vi "DAQ-WriteReadSine.vi"(0 "Maximum Input":dbl, 1 "Minimum Input":dbl, 5 "Physical Input Channel":tag, 7 "tiempo (s)":dbl, 9 "Amplitud":dbl, 11 "Frecuencia":dbl, 12 "Fs (S/s)":dbl, 13 "Minimum Output":dbl, 14 "Maximum Output":dbl, 15 "Physical Output Channel":tag) -> (4 "Vout":dbl, 6 "Output":dbl[](graph), 8 "Vin":dbl, 10 "Input":dbl[](graph))   [LabVIEW 2010]
uses:
  <vilib>/Utility/error.llb/DialogType.ctl
  <vilib>/DAQmx/write.llb/DAQmx Write (Analog DBL 1Chan 1Samp).vi
  <vilib>/DAQmx/read.llb/DAQmx Read (Analog DBL 1Chan 1Samp).vi
  <vilib>/DAQmx/create/channels.llb/DAQmx Create Channel (AO-Voltage-Basic).vi
  <vilib>/DAQmx/create/channels.llb/DAQmx Create Channel (AI-Voltage-Basic).vi
  <vilib>/daqmx/miscellaneous.llb/DAQmx Fill In Error Info.vi
  <vilib>/Analysis/NI_AALBase.lvlib
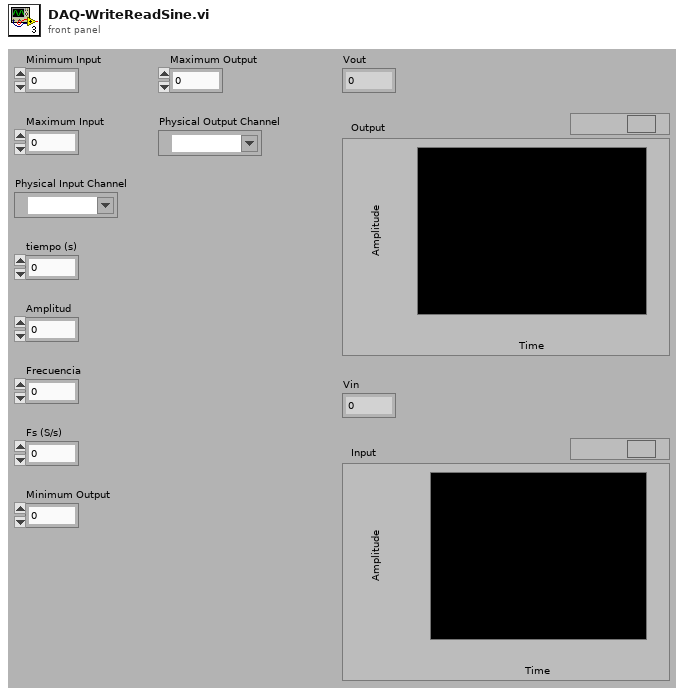
[diagram p1: front panel]
types:
  T1 = typedef "DialogType.ctl" = u16
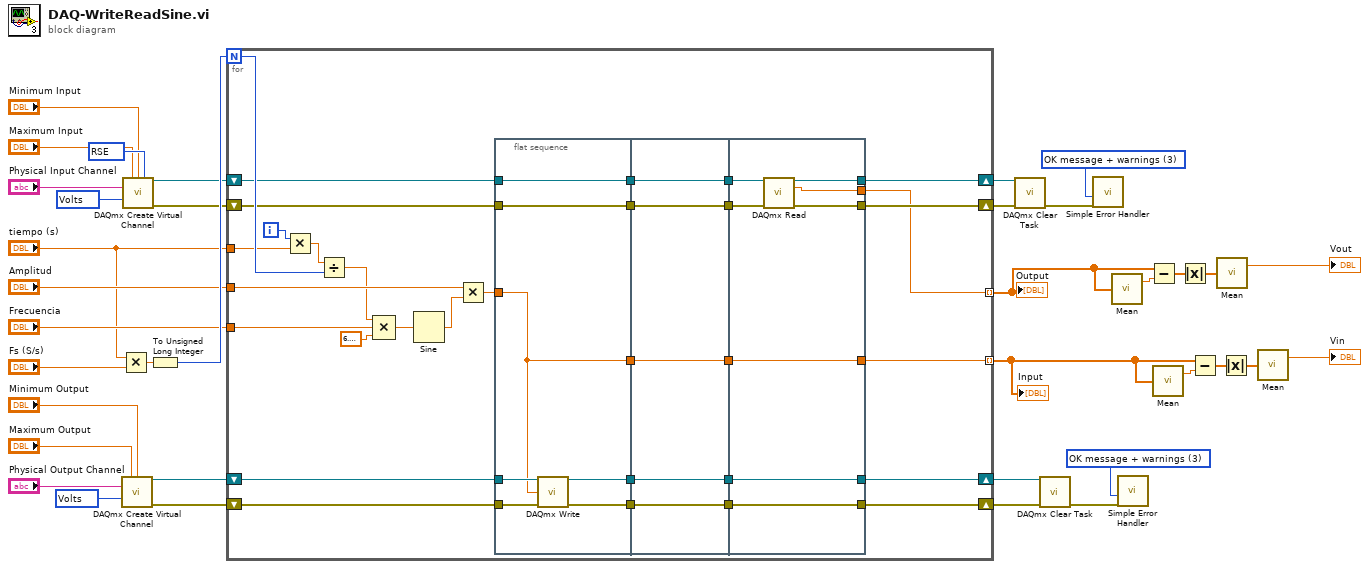
[diagram p0: block diagram]
diagram:
  w27 = 10083 items=["default"=-1, "RSE"=10083, "NRSE"=10078, "Differential"=10106, "Pseudodifferential"=12529] ("input terminal configuration")
  w17 = T1 3 items=["no dialog", "OK message", "continue or stop message", "OK message + warnings", "continue/stop + warnings"] ("type of dialog (OK msg:1)")
  w13 = T1 3 items=["no dialog", "OK message", "continue or stop message", "OK message + warnings", "continue/stop + warnings"] ("type of dialog (OK msg:1)")
  w5 = 10348 items=["Volts"=10348, "From Custom Scale"=10065] ("units")
  w1 = 10348 items=["Volts"=10348, "From Custom Scale"=10065] ("units")
  n1 = Multiply(x="tiempo (s)", y="Fs (S/s)") -> (x*y=w22:dbl)
  n2 = call-poly <vilib>:"DAQmx Create Virtual Channel.vi"("maximum value"="Maximum Output", "minimum value"="Minimum Output", "physical channels"="Physical Output Channel", "units"=w5) -> ("task out"=w9:refnum<k21>, "error out"=w10:errorcluster)  [unwired: 10 in]
  n3 = call-poly <vilib>:"DAQmx Create Virtual Channel.vi"("maximum value"="Maximum Input", "minimum value"="Minimum Input", "input terminal configuration"=w27, "physical channels"="Physical Input Channel", "units"=w1) -> ("task out"=w12:refnum<k21>, "error out"=w11:errorcluster)  [unwired: 9 in]
  n4 = To Unsigned Long Integer(number=w22) -> (unsigned 32bit integer=w26:u32)
  n5 = for {
    N: w26 -> [w63]
    shift-right: [w41] -> w15
    shift-left: w12 -> [w45]
    shift-right: [w40] -> w16
    shift-left: w11 -> [w42]
    shift-right: [w56] -> w19
    shift-left: w9 -> [w58]
    shift-right: [w55] -> w20
    shift-left: w10 -> [w57]
    tunnel: "tiempo (s)" -> [w59]
    tunnel: "Frecuencia" -> [w67]
    tunnel: "Amplitud" -> [w65]
    tunnel: [w54] -> w37 mode=indexing
    tunnel: [w39] -> w32 mode=indexing
    i -> [w60]
    n6 = Multiply(x=w60, y=w59) -> (x*y=w68:dbl)
    n7 = Divide(x=w68, y=w63) -> (x/y=w62:dbl)
    n8 = Compound Arithmetic op=MULTIPLY(w62, w67, 6.283185307179586) -> (w66:dbl)
    n9 = Sine(x=w66) -> (sin(x)=w64:dbl)
    n10 = Multiply(x=w65, y=w64) -> (x*y=w38:dbl)
    n11 = flat-sequence {
      tunnel: w58 -> [w75]
      tunnel: w57 -> [w74]
      tunnel: [w73] -> w53
      tunnel: [w72] -> w51
      tunnel: [w69] -> w49
      tunnel: [w71] -> w46
      tunnel: w45 -> [w71]
      tunnel: [w70] -> w43
      tunnel: w42 -> [w70]
      tunnel: w38 -> [w69]
      tunnel: w53 -> [w80]
      tunnel: [w80] -> w52
      tunnel: w51 -> [w79]
      tunnel: [w79] -> w50
      tunnel: w49 -> [w78]
      tunnel: [w78] -> w48
      tunnel: [w77] -> w47
      tunnel: w46 -> [w77]
      tunnel: [w76] -> w44
      tunnel: w43 -> [w76]
      tunnel: [w87] -> w55
      tunnel: [w88] -> w56
      tunnel: w52 -> [w88]
      tunnel: w50 -> [w87]
      tunnel: w48 -> [w86]
      tunnel: [w86] -> w54
      tunnel: w47 -> [w85]
      tunnel: w44 -> [w84]
      tunnel: [w83] -> w41
      tunnel: [w82] -> w40
      tunnel: [w81] -> w39
      frame #0 {
        n12 = call-poly <vilib>:"DAQmx Write.vi"("task/channels in"=w75, "data"=w69, "error in"=w74) -> ("task out"=w73:refnum<k21>, "error out"=w72:errorcluster)  [unwired: 10 in, 1 out]
      }
      frame #1 {
      }
      frame #2 {
        n13 = call-poly <vilib>:"DAQmx Read.vi"("task/channels in"=w85, "error in"=w84) -> ("task out"=w83:refnum<k21>, "data"=w81:dbl, "error out"=w82:errorcluster)  [unwired: 11 in]
      }
    }
  }
  "Output" <- w32
  "Input" <- w37
  n14 = call <vilib>:"DAQmx Clear Task.vi"("task in"=w15, "error in"=w16) -> ("error out"=w14:errorcluster)  [unwired: 13 in]
  n15 = call <vilib>:"DAQmx Clear Task.vi"("task in"=w19, "error in"=w20) -> ("error out"=w18:errorcluster)  [unwired: 13 in]
  n16 = call <vilib>:"Simple Error Handler.vi"("type of dialog (OK msg:1)"=w13, "error in (no error)"=w14) -> ()  [unwired: 3 in, 5 out]
  n17 = call <vilib>:"Mean.vi"("X"=w32) -> ("mean"=w31:dbl)  [unwired: 1 out]
  n18 = call <vilib>:"Simple Error Handler.vi"("type of dialog (OK msg:1)"=w17, "error in (no error)"=w18) -> ()  [unwired: 3 in, 5 out]
  n19 = Subtract(x=w32, y=w31) -> (x-y=w30:dbl[])
  n20 = call <vilib>:"Mean.vi"("X"=w37) -> ("mean"=w36:dbl)  [unwired: 1 out]
  n21 = Absolute Value(x=w30) -> (abs(x)=w29:dbl[])
  n22 = Subtract(x=w37, y=w36) -> (x-y=w35:dbl[])
  n23 = call <vilib>:"Mean.vi"("X"=w29) -> ("mean"=→"Vout":dbl)  [unwired: 1 out]
  n24 = Absolute Value(x=w35) -> (abs(x)=w34:dbl[])
  n25 = call <vilib>:"Mean.vi"("X"=w34) -> ("mean"=→"Vin":dbl)  [unwired: 1 out]
